vi "Save_Time_Traces.vi"() -> (5 "Plug in titles":string[](array[string]), 7 "Plug in values":string[](array[string]))   [LabVIEW 2012]
uses:
  Controls/Instrument_Array.ctl
  Globals/Meas_global.vi
panel:
  in  "Save Button":bool
  in  "No of desired samples/ch":i32
  in  "Down Sample":i32=1
  in  "File Extension":string=".xls"
  in  "Time Series":enum16{"Milliseconds", "Seconds"}(ring)
  in  "Full Header Info?":bool
  in  "Put each block into separate file":bool
  in  "Leave space between blocks?":bool
  in  "Precision":i16=6
  in  "Data to save":i32[](array[ring]) items=["Pitot (Ucal)", "HW (HF1)", "HW (HF2)", "HW (HF3)", "Gen (1101)", "Gen (1102)", "Gen (1103)", "Gen (1104)", "Gen (1105)", "Gen (1106)", "Gen (1107)", "Gen (1108)", "Gen (1201)", "Gen (1202)", "Gen (1203)", "Gen (1204)", "Gen (1205)", "Gen (1206)", "Gen (1301)", "Gen (1302)", "Gen (1303)", "Gen (1304)", "Gen (1305)", "Gen (1306)", "Gen (1307)", "Gen (1308)", "Gen (2101)", "Gen (2102)", "Gen (2103)", "Gen (2104)", "Gen (2201)", "Gen (2202)", "Gen (2203)", "Gen (2204)", "Gen (2301)", "Gen (2302)", "Gen (2303)", "Gen (2304)", "Gen (2401)", "Gen (2402)", "Gen (2403)", "Gen (2404)", "Gen (3101)", "Gen (3201)", "Gen (3202)", "Gen (3301)", "Gen (3302)", "Gen (3401)", "Gen (3402)", "Gen (3501)", "Gen (3502)", "Gen (3601)", "Gen (3602)", "Gen (3701)", "Gen (3702)", "Gen (3801)", "Gen (3802)", "Gen (3901)", "Gen (3902)", "Gen (3903)", "Gen (4101)", "Gen (4102)", "Gen (4103)", "Gen (4104)", "Gen (4105)", "Gen (4106)", "Gen (Quiet)", "Gen (Pref)", "Save Nothing"]
  in  "Separation Character":string="\t"
  # "WARNING! This VI has only been updated to work with ANALOGUE data at the moment!!"
  # "Run this VI to update the channel names"
  # "You Must have selected the \"Save Data\" option on the \nMeasurement Program for this vi to save time traces"
  # "0 means disabled"
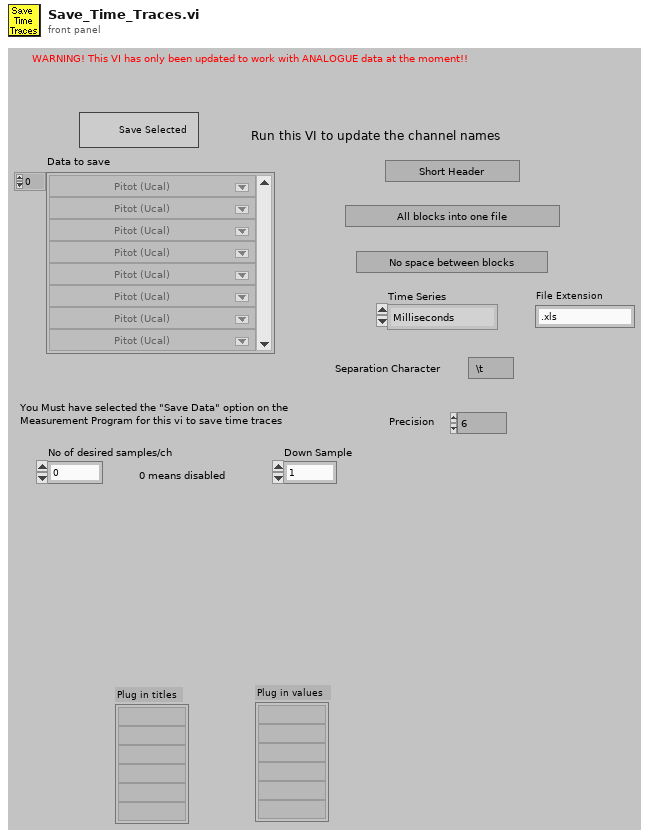
[diagram p1: front panel]
types:
  T1 = typedef "Analysis_info_cluster.ctl" = cluster{"Colour":u32, "Inst type":T2, "Inst name":string, "Symbol":string, "Code name":string, "Extra Info":string, "Inst Array":T3, "Extra Titles":string[], "Extra Values":string[], "U":dbl, "u^2":dbl, "u^3":dbl, "u^4":dbl, "Skew_u":dbl, "Kurt_u":dbl, "Sd Error in Mean":dbl, "% u'/U":dbl, "X":dbl, "Y":dbl, "Z":dbl, "Timescale integral to 25%":dbl, "Sd Error in Variance":dbl, "Calib File":path, "Calib Constants":dbl[], "Output Position":bool, "Full Stats":bool, "Av Sampling Rate":dbl, "Av No of Samples":dbl, "Total Meas Time (s)":dbl, "ADAM Ch Name":string}
  T2 = typedef "Inst_type.ctl" = enum16{"Propeller anemometer", "Raw voltage", "Pressure Transducer", "Pitot-static tube", "Preston tube", "Hot wire", "Cross wire 1", "Cross wire 2", "Generic Linear", "Generic Polynomial", "Generic BackPoly", "Fast FID", "Thermocouple", "Cold wire", "Pulsed Wire", "LDA Vel", "LDA Tran time", "LDA Arr time"}
  T3 = typedef "Instrument_Array.ctl" = enum16{"PWA", "LDA", "Analogue"}
  T4 = enum16{"Save no data", "Save data in new files", "Save data in existing files"}
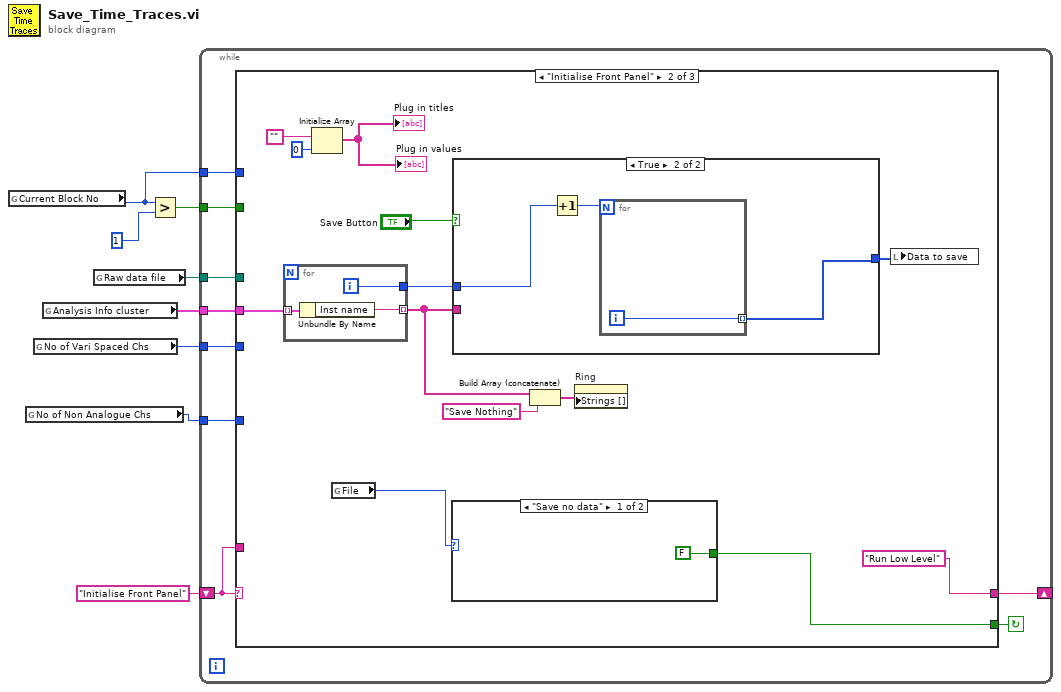
[diagram p0: block diagram]
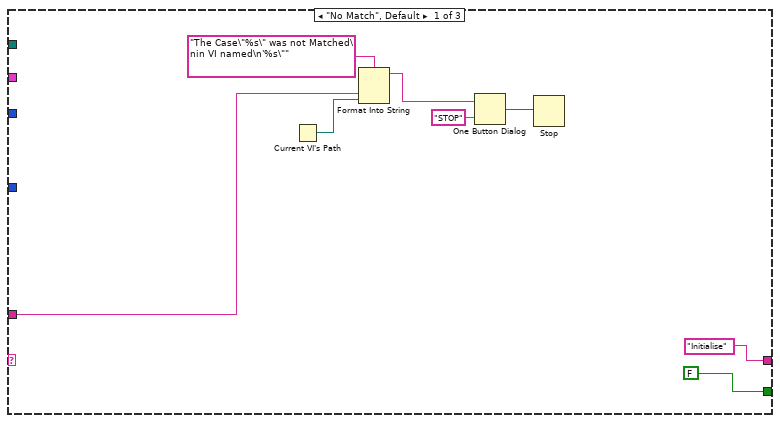
[diagram p2: hidden frame]
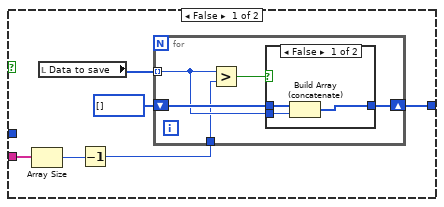
[diagram p3: hidden frame]
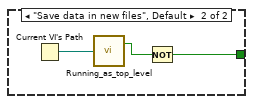
[diagram p5: hidden frame]
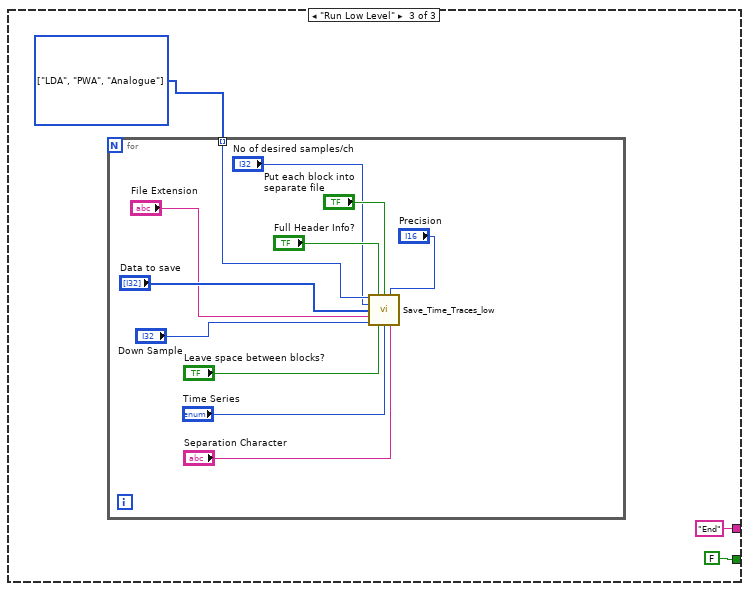
[diagram p6: hidden frame]
diagram:
  n1 = global read "Meas_global.vi" "Current Block No"() -> (w4:i32)
  n2 = global read "Meas_global.vi" "No of Non Analogue Chs"() -> (w1:i32)
  n3 = global read "Meas_global.vi" "No of Vari Spaced Chs"() -> (w2:i32)
  n4 = global read "Meas_global.vi" "Analysis Info cluster"() -> (w3:T1[])
  n5 = global read "Meas_global.vi" "Raw data file"() -> (w7:path)
  n6 = Greater?(x=w4, y=1) -> (0:w5:bool)
  n7 = while {
    shift-left: "Initialise Front Panel" -> [w15]
    shift-right: [w16] -> _
    tunnel: w7 -> [w14]
    tunnel: w5 -> [w13]
    tunnel: w4 -> [w12]
    tunnel: w3 -> [w11]
    tunnel: w2 -> [w10]
    tunnel: w1 -> [w9]
    stop <- w17 continue-if-true
    n8 = case shown="\"Initialise Front Panel\"" w15 {
      tunnel: [FALSE w28 FALSE] -> w17
      tunnel: ["Initialise" "Run Low Level" ("t") "End" ("t")] -> w16
      tunnel: w15 -> [w20 _ _]
      tunnel: w14 -> [_ _ _]
      tunnel: w13 -> [_ _ _]
      tunnel: w12 -> [_ _ _]
      tunnel: w11 -> [_ w35 _]
      tunnel: w10 -> [_ _ _]
      tunnel: w9 -> [_ _ _]
      frame "No Match", Default {
        n9 = Current VI's Path() -> (path=w19:path)
        n10 = Format Into String(format string="The Case\"%s\" was not Matched\nin VI named\n'%s\"" ("Format String"), w20, w19) -> (resulting string=w23:string)  [unwired: 2 in, 1 out]
        n11 = One Button Dialog(message=w23, button name ("OK")="STOP") -> (true=w21:bool)
        n12 = Stop(stop? (T)=w21) -> ()
      }
      frame "Initialise Front Panel" {
        n13 = for {
          tunnel: w35 -> [w64] mode=indexing
          tunnel: [w63] -> w31 mode=indexing
          tunnel: [w62] -> w26
          i -> [w62]
          n14 = Unbundle By Name(w64) -> ("Inst name"=w63:string)
        }
        n15 = Initialize Array("", 0) -> (→"Plug in values" →"Plug in titles":string[])
        n16 = global read "Meas_global.vi" "File"() -> (w29:T4)
        n17 = case shown="\"Save no data\"" w29 {
          tunnel: [FALSE w59] -> w28
          frame "Save no data" {
          }
          frame "Save data in new files", Default {
            n18 = Current VI's Path() -> (path=w60:path)
            n19 = call "Running_as_top_level.vi"("Vi path name"=w60) -> ("Top Level"=w61:bool)  [unwired: 1 out]
            n20 = Not(x=w61) -> (.not. x?=w59:bool)
          }
        }
        n21 = case shown="True" "Save Button" {
          tunnel: [w42 w55] -> w34
          tunnel: w31 -> [w39 _]
          tunnel: w26 -> [_ w56]
          frame False {
            n22 = Array Size(array=w39) -> (size(s)=w41:i32)
            n23 = local read "Data to save"() -> (w44:i32[])
            n24 = Decrement(x=w41) -> (x-1=w40:i32)
            n25 = for {
              tunnel: w44 -> [w46] mode=indexing
              shift-right: [w47] -> w42
              shift-left: i32[] [] -> [w48]
              tunnel: w40 -> [w45]
              n26 = Greater?(x=w46, y=w45) -> (0:w49:bool)
              n27 = case shown="False" w49 {
                tunnel: w48 -> [w52 w53]
                tunnel: [w51 w53] -> w47
                tunnel: w46 -> [w50 _]
                frame False {
                  n28 = Build Array (concatenate)(w52, w50) -> (w51:i32[])
                }
                frame True {
                }
              }
            }
          }
          frame True {
            n29 = Increment(x=w56) -> (x+1=w54:i32)
            n30 = for {
              N: w54 -> [_]
              tunnel: [w57] -> w55 mode=indexing
              i -> [w57]
            }
          }
        }
        n31 = Build Array (concatenate)(w31, "Save Nothing") -> (w32:string[])
        n32 = property on="Ring" class="Ring (strict)"("Strings []"=w32) -> ()  [unwired: 2 in, 2 out]
        n33 = local write "Data to save"(w34) -> ()
      }
      frame "Run Low Level" {
        w66 = T3[] [enum."LDA", enum."PWA", enum."Analogue"] items=["PWA", "LDA", "Analogue"]
        n34 = for {
          tunnel: w66 -> [w71] mode=indexing
          n35 = call "Save_Time_Traces_low.vi"("Data Type"=w71, "Full Header Info?"="Full Header Info?", "Put each block into separate file"="Put each block into separate file", "Precision"="Precision", "No of desired samples/ch"="No of desired samples/ch", "Data to save"="Data to save", "File Extension"="File Extension", "Down Sample"="Down Sample", "Leave space between blocks?"="Leave space between blocks?", "Time Series"="Time Series", "Separation Character"="Separation Character") -> ()  [unwired: 5 out]
        }
      }
    }
  }
